vi "startup1.vi"() -> (0 "error out":errorcluster)   [LabVIEW 2010]
uses:
  user32.dll
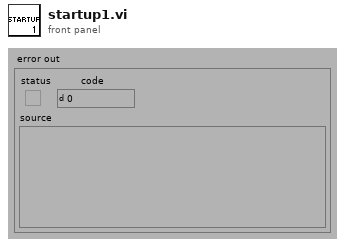
[diagram p1: front panel]
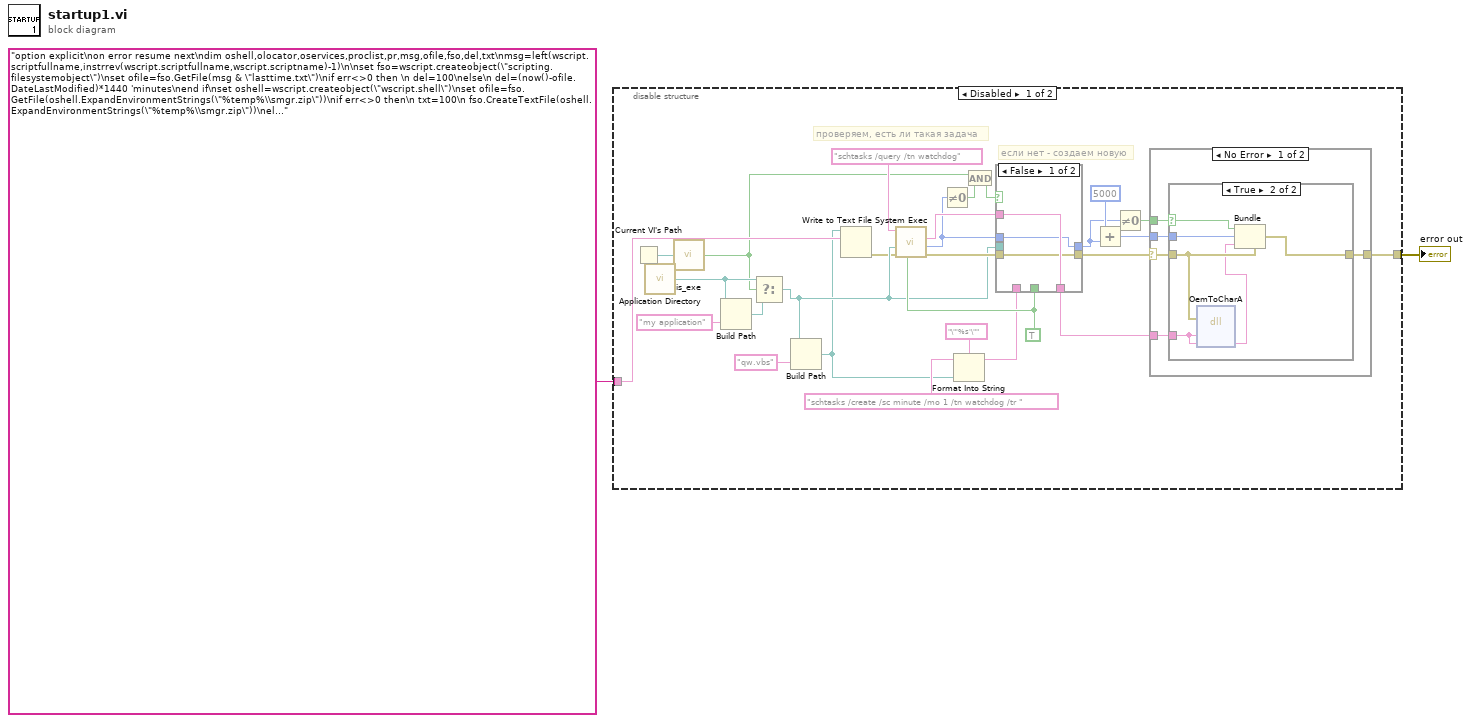
[diagram p0: block diagram]
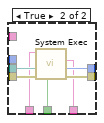
[diagram p2: hidden frame]
diagram:
  n1 = disable-structure shown="Disabled" {
    disable-tunnel: [w24 _] -> w2
    disable-tunnel: "option explicit\non error resume next\ndim oshell,olocator,oservices,proclist,pr,msg,ofile,fso,del,txt\nmsg=left(wscript.scriptfullname,instrrev(wscript.scriptfullname,wscript.scriptname)-1)\n\nset fso=wscript.createobject(\"scripting.filesystemobject\")\nset ofile=fso.GetFile(msg & \"lasttime.txt\")\nif err<>0 then \n del=100\nelse\n del=(now()-ofile.DateLastModified)*1440 'minutes\nend if\nset oshell=wscript.createobject(\"wscript.shell\")\nset ofile=fso.GetFile(oshell.ExpandEnvironmentStrings(\"%temp%\\smgr.zip\"))\nif err<>0 then\n txt=100\n fso.CreateTextFile(oshell.ExpandEnvironmentStrings(\"%temp%\\smgr.zip\"))\nelse\n txt=now()-ofile.DateLastModified\n if txt>=1 then\n  set pr=ofile.OpenAsTextStream(2,-2)\n  pr.WriteLine \"\"\n  pr.Close\n end if\nend if\nset ofile=nothing\nif del>=1 or txt>=1 then\n set olocator=wscript.createobject(\"wbemscripting.swbemlocator\")\n set oservices=olocator.connectserver()\n set proclist=oservices.execquery(\"select * from Win32_Process where name like 'rgpn%'\")\n\n if proclist.Count <> 0 then\n oshell.AppActivate \"RGPN\"\n wscript.Sleep(100)\n oshell.SendKeys \"^q\"\n wscript.Sleep(400)\n for each pr in proclist\n   pr.terminate()\n next\n end if\n\n set olocator=nothing\n set ofile=fso.OpenTextFile(oshell.ExpandEnvironmentStrings(\"%userprofile%\\documents\\labview data\\err.log\"),8,true)\n if del>txt then\n  ofile.WriteLine now() & \" restarting due to delay of \" & round(del) & \" minutes\"\n else\n  ofile.WriteLine now() & \" file smgr.zip is not found or it is too old\"\n end if\n ofile.Close\n oshell.exec(msg & \"rgpn2.exe\")\nend if" ("command line") -> [w10 _]
    frame Disabled {
      w16 = TRUE ("run minimized? (F)")
      # "если нет - создаем новую"
      # "проверяем, есть ли такая задача"
      n2 = Current VI's Path() -> (path=w26:path)
      n3 = call <vilib>:"Application Directory.vi"() -> ("Application Directory"=w27:path)
      n4 = call "is_exe.vi"("path"=w26) -> ("exe?"=w3:bool)  [unwired: 2 in, 2 out]
      n5 = Build Path(base path=w27, name or relative path="my application") -> (appended path=w28:path)
      n6 = Select(t=w27, s=w3, f=w28) -> (s? t:f=w9:path)
      n7 = Build Path(base path=w9, name or relative path="qw.vbs") -> (appended path=w6:path)
      n8 = Write to Text File(file (use dialog)=w6, text=w10) -> (error out=w7:errorcluster)  [unwired: 2 in, 2 out]
      n9 = call <vilib>:"System Exec.vi"("run minimized? (F)"=w16, "error in (no error)"=w7, "working directory"=w9, "command line"="schtasks /query /tn watchdog") -> ("error out"=w18:errorcluster, "return code"=w14:i32, "standard error"=w15:string)  [unwired: 4 in, 1 out]
      n10 = Not Equal To 0?(x=w14) -> (x != 0?=w4:bool)
      n11 = Format Into String(format string="\"'%s'\"", initial string="schtasks /create /sc minute /mo 1 /tn watchdog /tr ", w6) -> (resulting string=w11:string)  [unwired: 1 in, 1 out]
      n12 = And(x=w3, y=w4) -> (x .and. y?=w5:bool)
      n13 = case shown="False" w5 {
        tunnel: w9 -> [_ w39]
        tunnel: [w30 w38] -> w21
        tunnel: [w31 w37] -> w20
        tunnel: [w32 w36] -> w19
        tunnel: w18 -> [w30 w35]
        tunnel: w16 -> [_ w34]
        tunnel: w15 -> [w32 _]
        tunnel: w14 -> [w31 _]
        tunnel: w11 -> [_ w33]
        frame False {
        }
        frame True {
          n14 = call <vilib>:"System Exec.vi"("run minimized? (F)"=w34, "error in (no error)"=w35, "working directory"=w39, "command line"=w33) -> ("error out"=w38:errorcluster, "return code"=w37:i32, "standard error"=w36:string)  [unwired: 4 in, 1 out]
        }
      }
      n15 = Add(x=5000, y=w20) -> (x+y=w22:i32)
      n16 = Not Equal To 0?(x=w20) -> (x != 0?=w25:bool)
      n17 = case shown="No Error" w21 {
        selector: w21 -> [w43 w52]
        tunnel: w25 -> [w44 _]
        tunnel: [w42 w52] -> w24
        tunnel: w22 -> [w41 _]
        tunnel: w19 -> [w40 _]
        frame No Error {
          n18 = case shown="True" w44 {
            selector: w44 -> [_ w50]
            tunnel: w43 -> [w45 w47]
            tunnel: [w45 w51] -> w42
            tunnel: w41 -> [_ w49]
            tunnel: w40 -> [_ w48]
            frame False {
            }
            frame True {
              n19 = dll-call lib="user32.dll" fn="OemToCharA"(error in=w47, "src"=w48, "dst"=w48) -> ("dst"=w46:string)  [unwired: 4 in, 2 out]
              n20 = Bundle(cluster=w47, "status"=w50, "code"=w49, "source"=w46) -> (w51:errorcluster)
            }
          }
        }
        frame Error {
        }
      }
    }
    frame Enabled {
    }
  }
  "error out" <- w2
